vi "Write target.vi"(8 "error in (no error)":errorcluster, 10 "TCSGuiderStatus.lvlib:GWTargetPositionParameters.lvclass":refnum<class "GWTargetPositionParameters.lvclass">, 11 "WaveFrontTargetPosition in":refnum<class "WaveFrontTargetPosition.lvclass">) -> (0 "error out":errorcluster, 3 "WaveFrontTargetPosition out":refnum<class "WaveFrontTargetPosition.lvclass">)   [LabVIEW 2014, in "TCSDataDefinitions.lvlib" / "TCSWFSStatus.lvlib" / "WaveFrontTargetPosition.lvclass"]
uses:
  WaveFrontTargetPosition.lvclass
  TCSGuiderStatus/GWTargetPositionParameters/GWTargetPositionParameters.lvclass
  WaveFrontTargetPosition.lvclass/WaveFrontTargetPosition.ctl
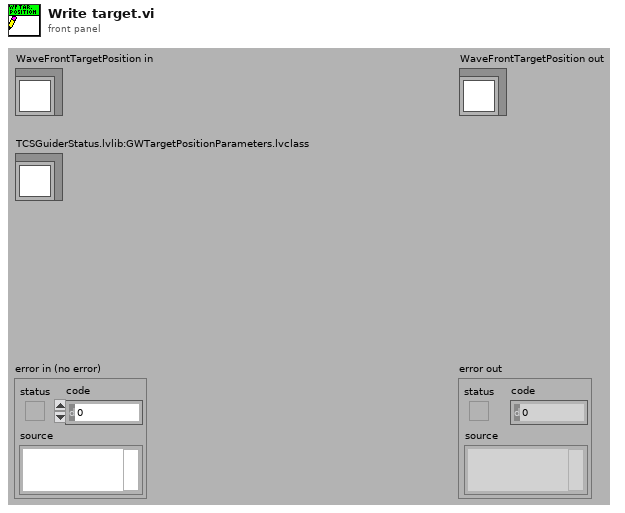
[diagram p1: front panel]
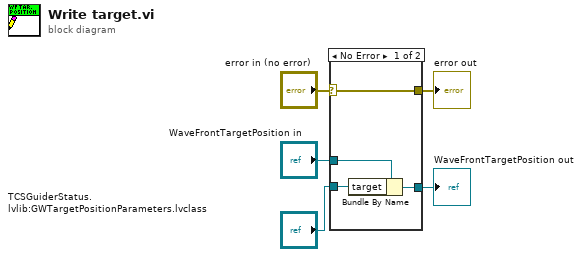
[diagram p0: block diagram]
diagram:
  n1 = case shown="No Error" "error in (no error)" {
    selector: "error in (no error)" -> [w9 w10]
    tunnel: [w9 w10] -> w4
    tunnel: [w7 w11] -> w2
    tunnel: "WaveFrontTargetPosition in" -> [w8 w11]
    tunnel: "TCSGuiderStatus.lvlib:GWTargetPositionParameters.lvclass" -> [w6 _]
    frame No Error {
      n2 = Bundle By Name(cluster=w8, "target"=w6) -> (w7:refnum<class "WaveFrontTargetPosition.lvclass">)
    }
    frame Error {
    }
  }
  "error out" <- w4
  "WaveFrontTargetPosition out" <- w2
